vi "Puff_release3.vi"() -> (5 "Plug in titles":string[](array[string]), 7 "Plug in values":string[](array[string]))   [LabVIEW 2010]
uses:
  Controls/Post_Process.ctl
  Globals/Plug_in_data_global.vi
  Globals/Meas_global.vi
  Globals/Constants_global.vi
  Globals/Dynamic_call_global.ph.vi
  <vilib>/Analysis/NI_AALPro.lvlib
panel:
  in  "Save JPG images":bool
  out "delay":dbl format="%.2f"
  out "Pulse Width":dbl format="%.2f"
  out "falltime":dbl format="%.2f"
  out "top":dbl format="%.2f"
  out "risetime":dbl format="%.2f"
  in  "Save Time pdf?":bool
  out "Pdf":cluster{"Axis":dbl[], dbl[]}(graph)
  in  "Histogram Time":dbl format="%.2f"
  out "Current Block No":i32
  in  "Save averaged traces?":bool
  in  "Save Block Time Trace?":bool
  in  "Pause Mode":T1(ring)
  in  "OK":bool
  out "No of Valid Blocks":dbl
  out "Valve Trace":cluster{dbl, dbl, dbl[]}(graph)
  out "FFID Trace":cluster{dbl, dbl, dbl[]}(graph)
  out "Source On":i32
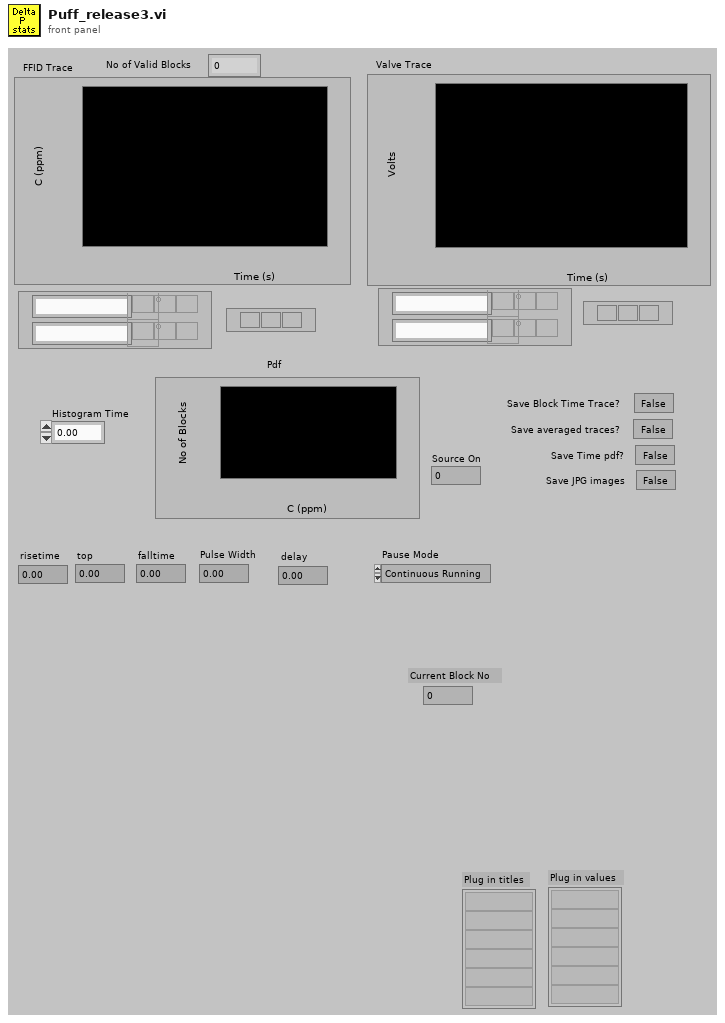
[diagram p1: front panel]
types:
  T1 = enum16{"Continuous Running", "After Each  Block"}
  T2 = typedef "Post_Process.ctl" = enum16{"Take New Data", "Post Process Raw Data File"}
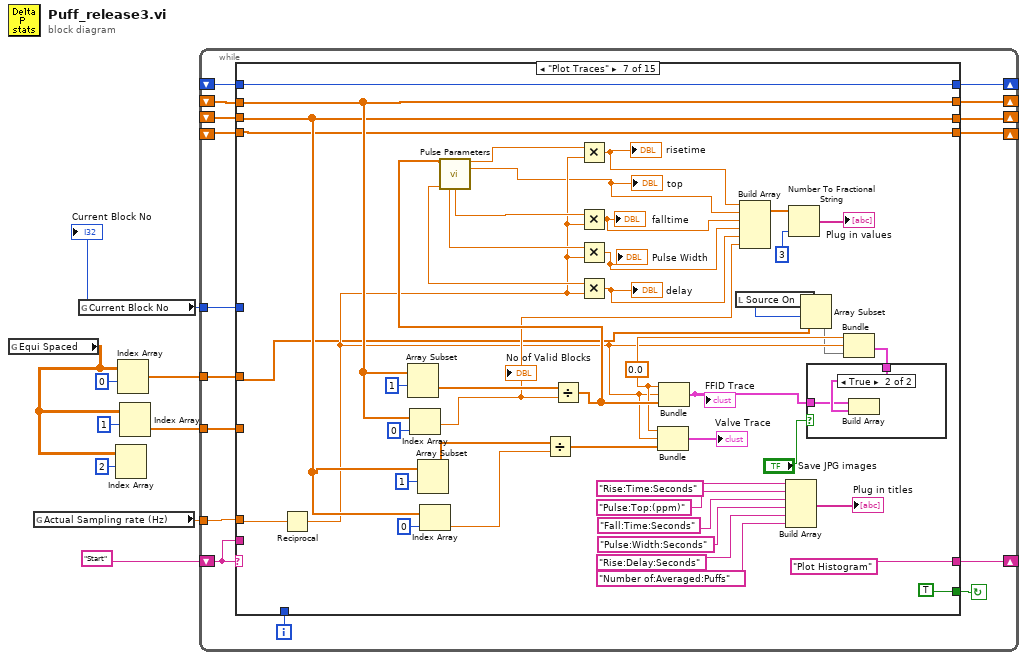
[diagram p0: block diagram]
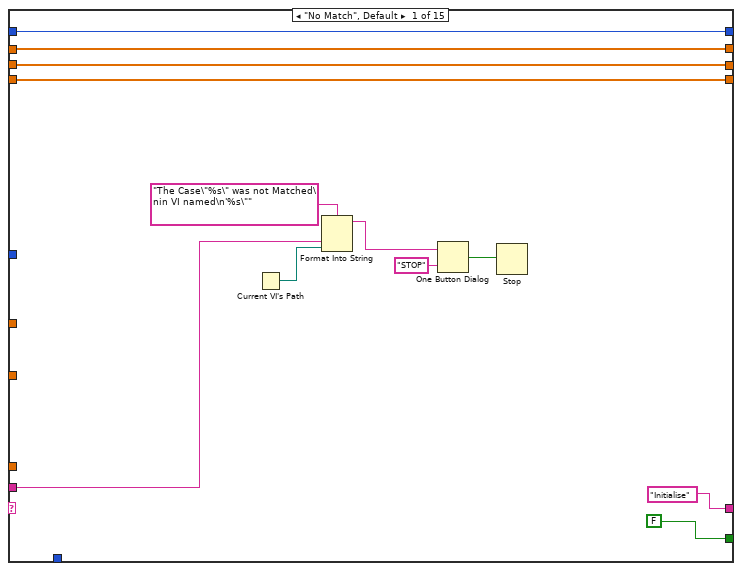
[diagram p2: hidden frame]
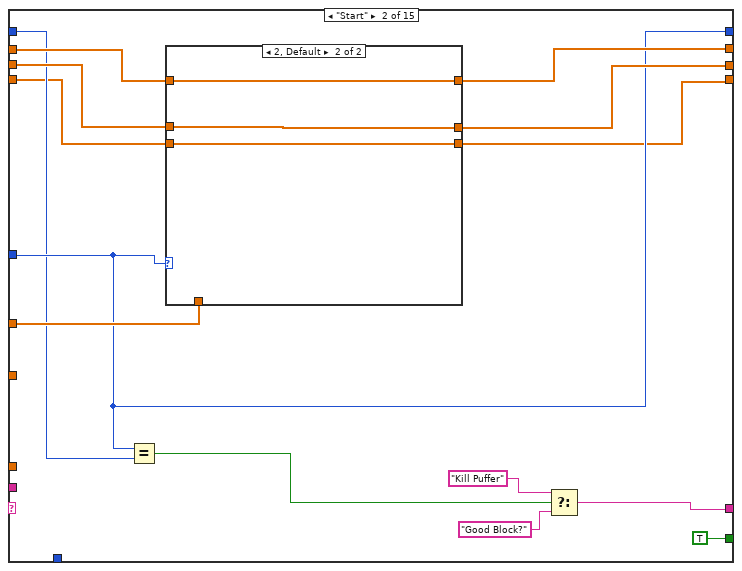
[diagram p3: hidden frame]
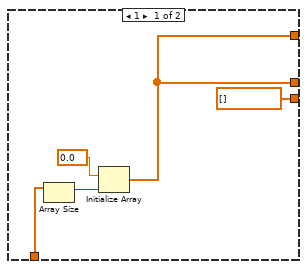
[diagram p4: hidden frame]
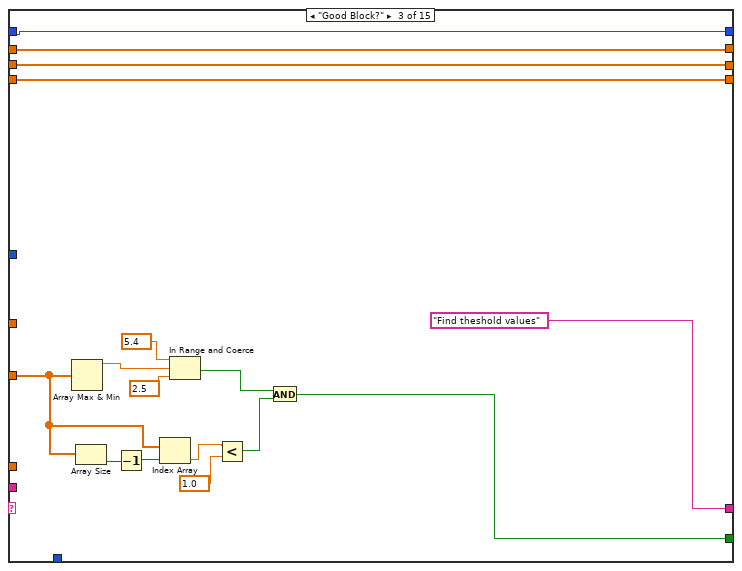
[diagram p5: hidden frame]
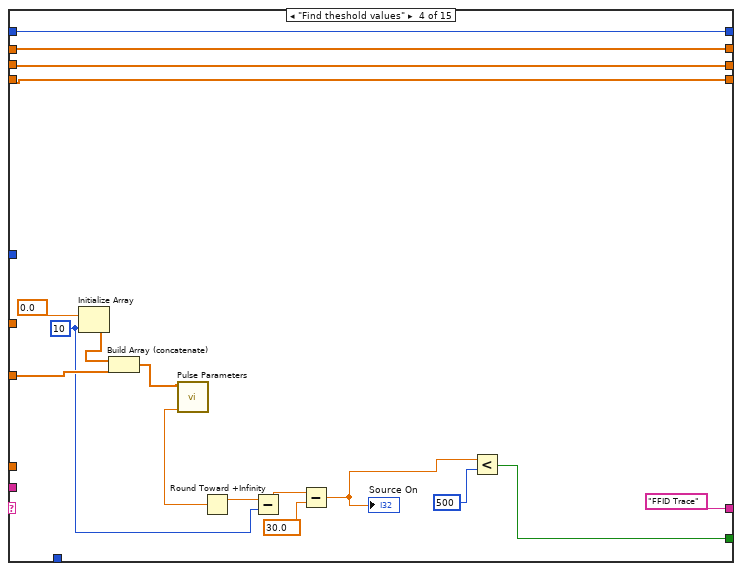
[diagram p6: hidden frame]
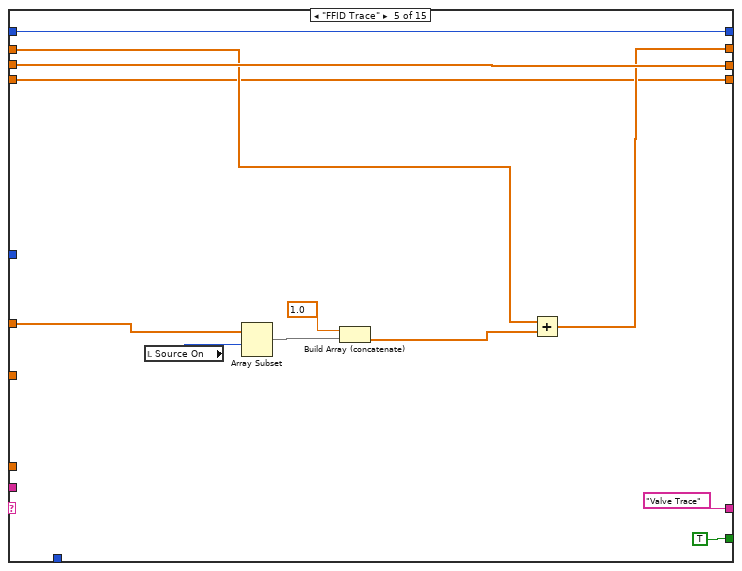
[diagram p7: hidden frame]
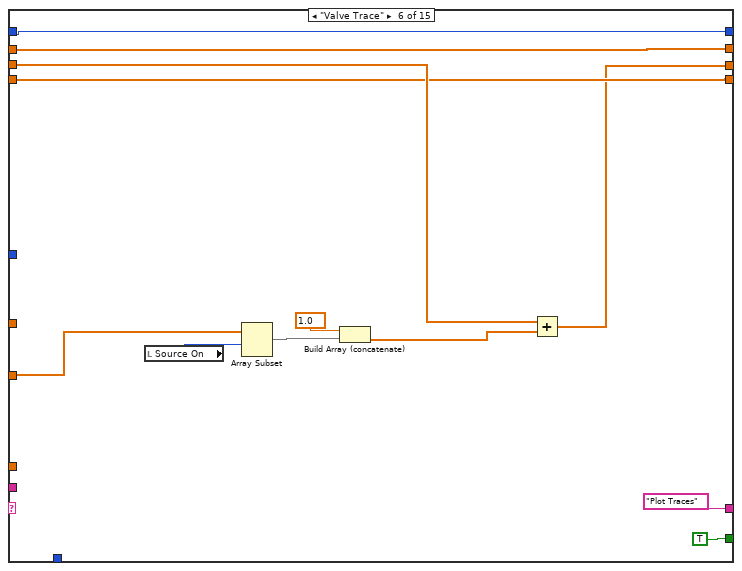
[diagram p8: hidden frame]
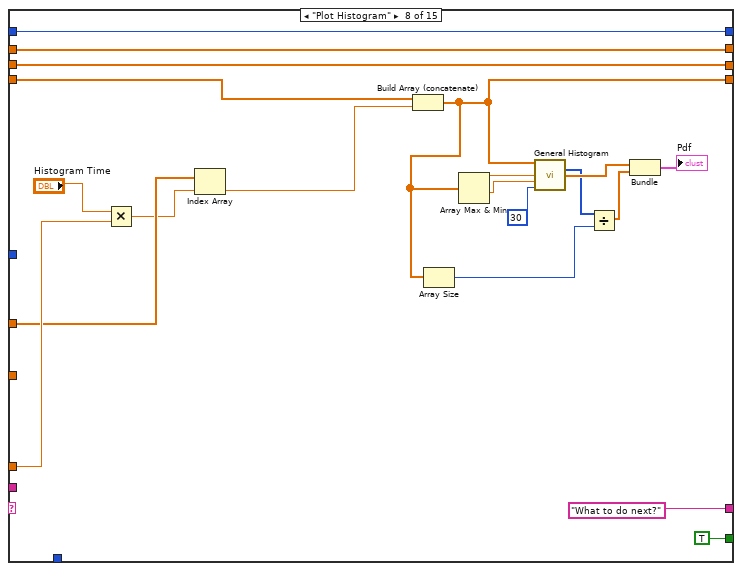
[diagram p10: hidden frame]
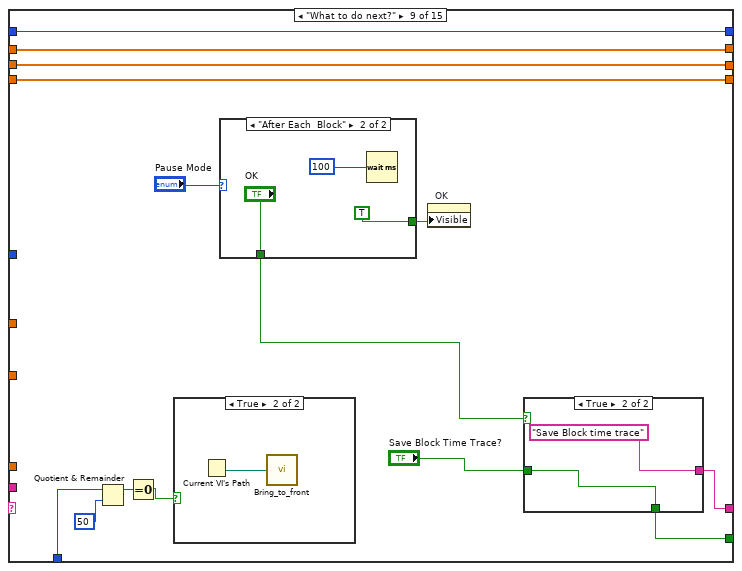
[diagram p11: hidden frame]
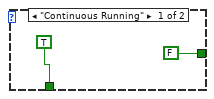
[diagram p13: hidden frame]
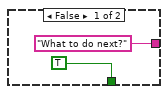
[diagram p14: hidden frame]
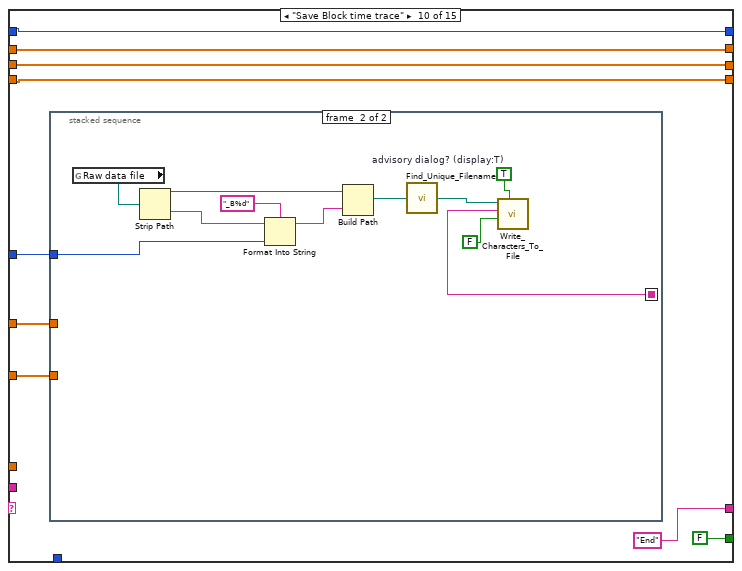
[diagram p15: hidden frame]
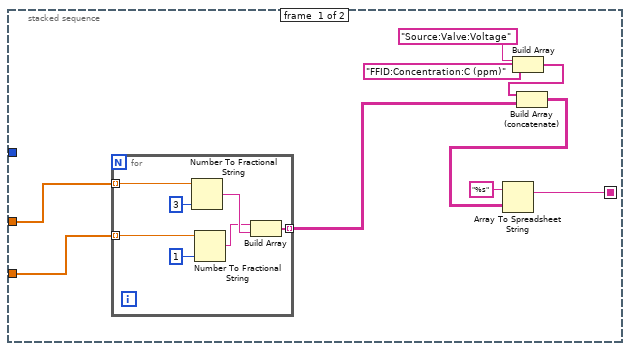
[diagram p16: hidden frame]
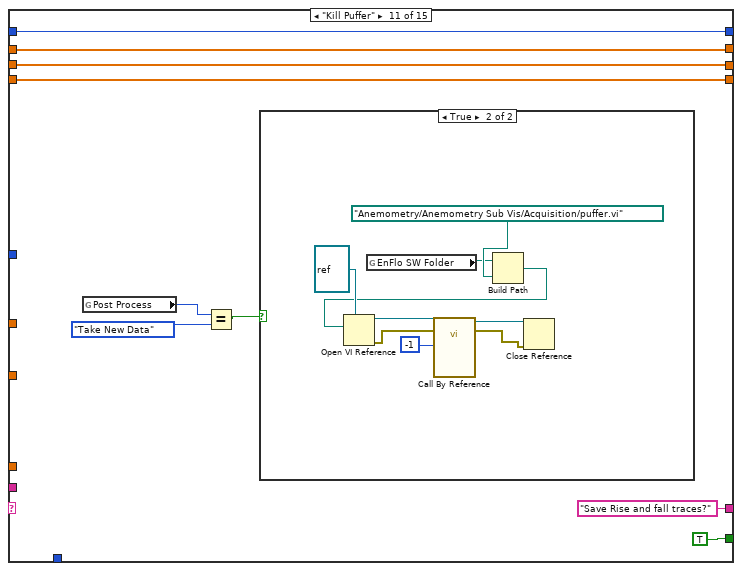
[diagram p17: hidden frame]
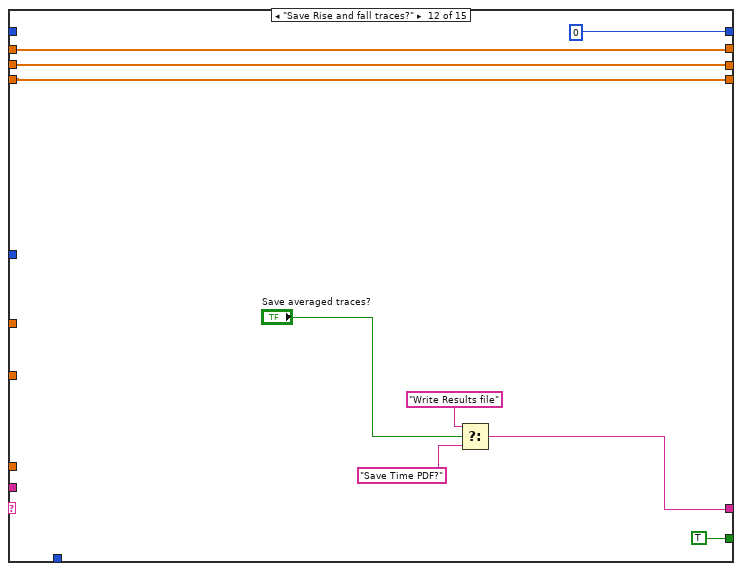
[diagram p19: hidden frame]
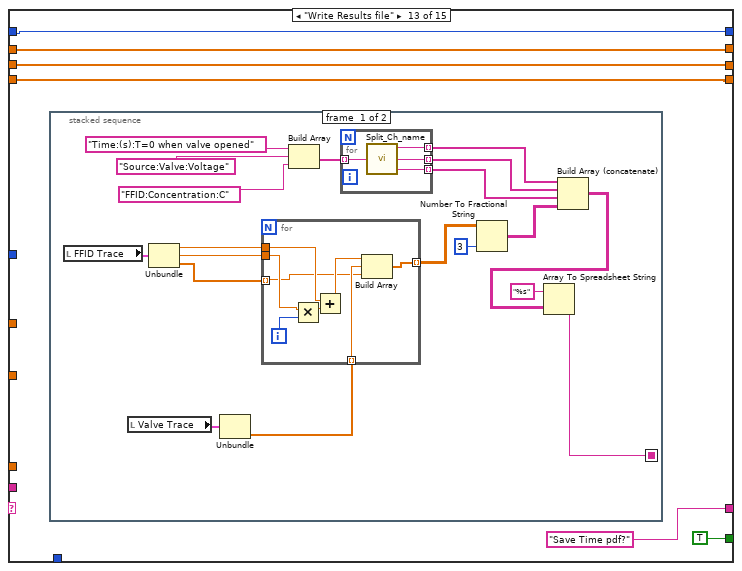
[diagram p20: hidden frame]
diagram:
  n1 = global read "Plug_in_data_global.vi" "Equi Spaced"() -> (w1:dbl[][])
  n2 = global read "Meas_global.vi" "Actual Sampling rate (Hz)"() -> (w5:dbl)
  n3 = global read "Meas_global.vi" "Current Block No"() -> (w4:i32)
  "Current Block No" <- w4
  n4 = Index Array(array=w1, index (row)=2) -> ()  [unwired: 1 in, 1 out]
  n5 = Index Array(array=w1, index (row)=0) -> (element=w6:dbl[])  [unwired: 1 in]
  n6 = Index Array(array=w1, index (row)=1) -> (element=w7:dbl[])  [unwired: 1 in]
  n7 = while {
    shift-left: "Start" -> [w23]
    shift-right: [w24] -> _
    shift-right: [w22] -> _
    shift-left: _ -> [w19]
    shift-right: [w21] -> _
    shift-left: _ -> [w20]
    tunnel: w7 -> [w18]
    tunnel: w6 -> [w17]
    tunnel: w5 -> [w16]
    tunnel: w4 -> [w15]
    shift-right: [w12] -> _
    shift-left: _ -> [w13]
    shift-right: [w10] -> _
    shift-left: _ -> [w11]
    i -> [w14]
    stop <- w25 continue-if-true
    n8 = case shown="\"Plot Traces\"" w23 {
      tunnel: [FALSE TRUE ("Processing last block?") w63 w88 TRUE ("Processing last block?") TRUE ("Processing last block?") TRUE ("Processing last block?") TRUE ("Processing last block?") w186 FALSE ("Processing last block?") TRUE ("Processing last block?") TRUE ("Processing last block?") TRUE ("Processing last block?") "Save Time pdf?" FALSE ("Processing last block?")] -> w25
      tunnel: ["Initialise" w41 "Find theshold values" "FFID Trace" "Valve Trace" "Plot Traces" "Plot Histogram" ("f") "What to do next?" ("f") w194 "End" "Save Rise and fall traces?" w263 "Save Time pdf?" "Save Time pdf" "End"] -> w24
      tunnel: w23 -> [w32 _ _ _ _ _ _ _ _ _ _ _ _ _ _]
      tunnel: [w29 w50 w75 w91 w100 w110 w159 w183 w197 w216 w252 w270 w276 w340 w349] -> w22
      tunnel: [w28 w48 w74 w90 w102 w105 w155 w182 w196 w215 w251 w269 w275 w339 w348] -> w21
      tunnel: w20 -> [w28 w47 w74 w90 w102 w109 w155 w182 w196 w215 w251 w269 w275 w339 w348]
      tunnel: w19 -> [w29 w49 w75 w91 w99 w110 w159 w183 w197 w216 w252 w270 w276 w340 w349]
      tunnel: w18 -> [_ _ w71 w84 _ w111 _ _ _ w212 _ _ _ _ w345]
      tunnel: w17 -> [_ w46 _ _ w101 _ w126 w178 _ w211 _ _ _ _ w344]
      tunnel: w16 -> [_ _ _ _ _ _ w151 w179 _ _ _ _ _ _ _]
      tunnel: w15 -> [_ w45 _ _ _ _ _ _ _ w210 _ _ _ _ w343]
      tunnel: w14 -> [_ _ _ _ _ _ _ _ w191 _ _ _ _ _ _]
      tunnel: w13 -> [w27 w44 w64 w87 w94 w108 w147 w181 w187 w209 w248 _ w272 _ w342]
      tunnel: [w27 w45 w64 w87 w94 w108 w147 w181 w187 w209 w248 0 w272 0 w342] -> w12
      tunnel: w11 -> [w26 w38 w62 w79 w93 w106 w130 w175 w184 w208 w244 w267 w271 w336 w341]
      tunnel: [w26 w39 w62 w79 w93 w106 w130 w167 w184 w208 w244 w267 w271 w336 w341] -> w10
      frame "No Match", Default {
        n9 = Current VI's Path() -> (path=w31:path)
        n10 = Format Into String(format string="The Case\"%s\" was not Matched\nin VI named\n'%s\"" ("Format String"), w32, w31) -> (resulting string=w35:string)  [unwired: 2 in, 1 out]
        n11 = One Button Dialog(message=w35, button name ("OK")="STOP") -> (true=w33:bool)
        n12 = Stop(stop? (T)=w33) -> ()
      }
      frame "Start" {
        n13 = Equal?(x=w45, y=w44) -> (x = y?=w43:bool)
        n14 = case shown="2, Default" w45 {
          tunnel: [w53 w59] -> w50
          tunnel: w49 -> [_ w59]
          tunnel: [w53 w58] -> w48
          tunnel: w47 -> [_ w58]
          tunnel: w46 -> [w56 _]
          tunnel: [dbl[] [] w57] -> w39
          tunnel: w38 -> [_ w57]
          frame 1 {
            n15 = Array Size(array=w56) -> (size(s)=w55:i32)
            n16 = Initialize Array(0.0 ("element"), w55) -> (w53:dbl[])
          }
          frame 2, Default {
          }
        }
        n17 = Select(t="Kill Puffer", s=w43, f="Good Block?") -> (s? t:f=w41:string)
      }
      frame "Good Block?" {
        n18 = Array Max & Min(array=w71) -> (max value=w61:dbl)  [unwired: 3 out]
        n19 = Array Size(array=w71) -> (size(s)=w70:i32)
        n20 = Decrement(x=w70) -> (x-1=w69:i32)
        n21 = Index Array(array=w71, index=w69) -> (element=w68:dbl)
        n22 = In Range and Coerce(upper limit=5.4, x=w61, lower limit=2.5 ("y")) -> (In Range?=w65:bool)  [unwired: 1 out]
        n23 = Less?(x=w68, y=1.0) -> (x < y?=w66:bool)
        n24 = And(x=w65, y=w66) -> (x .and. y?=w63:bool)
      }
      frame "Find theshold values" {
        w80 = 10 ("dimension size")
        n25 = Initialize Array(0.0, w80) -> (w83:dbl[])
        n26 = Build Array (concatenate)(w83, w84) -> (w85:dbl[])
        n27 = call <vilib>:"Pulse Parameters.vi"("X"=w85) -> ("delay"=w82:dbl)  [unwired: 4 in, 10 out]
        n28 = Round Toward +Infinity(x=w82) -> (ceil(x): smallest int >= x=w81:dbl)
        n29 = Subtract(x=w81, y=w80) -> (x-y=w78:dbl)
        n30 = Subtract(x=w78, y=30.0) -> (x-y=w76:dbl)
        "Source On" <- w76
        n31 = Less?(x=w76, y=500) -> (x < y?=w88:bool)
      }
      frame "FFID Trace" {
        n32 = local read "Source On"() -> (w96:i32)
        n33 = Array Subset(array=w101, index=w96) -> (w95:dbl[])  [unwired: 1 in]
        n34 = Build Array (concatenate)(1.0, w95) -> (w97:dbl[])
        n35 = Add(x=w99, y=w97) -> (x+y=w100:dbl[])
      }
      frame "Valve Trace" {
        n36 = local read "Source On"() -> (w113:i32)
        n37 = Array Subset(array=w111, index=w113) -> (w112:dbl[])  [unwired: 1 in]
        n38 = Build Array (concatenate)(1.0, w112) -> (w114:dbl[])
        n39 = Add(x=w109, y=w114) -> (x+y=w105:dbl[])
      }
      frame "Plot Traces" {
        w129 = 0.0
        n40 = Reciprocal(x=w151) -> (1/x=w128:dbl)
        n41 = Array Subset(array=w159, index=1) -> (w158:dbl[])  [unwired: 1 in]
        n42 = Index Array(array=w159, index=0) -> (element=w138:dbl)
        "No of Valid Blocks" <- w138
        n43 = Array Subset(array=w155, index=1) -> (w154:dbl[])  [unwired: 1 in]
        n44 = Index Array(array=w155, index=0) -> (element=w153:dbl)
        n45 = Divide(x=w154, y=w153) -> (x/y=w149:dbl[])
        n46 = Divide(x=w158, y=w138) -> (x/y=w146:dbl[])
        n47 = call <vilib>:"Pulse Parameters.vi"("X"=w146) -> ("risetime"=w145:dbl, "top"=w122:dbl, "delay"=w142:dbl, "duration"=w143:dbl, "falltime"=w144:dbl)  [unwired: 4 in, 6 out]
        "top" <- w122
        n48 = Multiply(x=w145, y=w128) -> (x*y=w121:dbl)
        "risetime" <- w121
        n49 = Multiply(x=w144, y=w128) -> (x*y=w120:dbl)
        "falltime" <- w120
        n50 = Multiply(x=w143, y=w128) -> (x*y=w119:dbl)
        "Pulse Width" <- w119
        n51 = Multiply(x=w142, y=w128) -> (x*y=w118:dbl)
        "delay" <- w118
        n52 = Bundle(w129, w128, w149) -> (→"Valve Trace":cluster{dbl, dbl, dbl[]})  [unwired: 1 in]
        n53 = Bundle(w129, w128, w146) -> (w123:cluster{dbl, dbl, dbl[]})  [unwired: 1 in]
        "FFID Trace" <- w123
        n54 = local read "Source On"() -> (w127:i32)
        n55 = Build Array(w121, w122, w120, w119, w118, w138) -> (w141:dbl[])
        n56 = Build Array("Rise:Time:Seconds", "Pulse:Top:(ppm)", "Fall:Time:Seconds", "Pulse:Width:Seconds", "Rise:Delay:Seconds", "Number of:Averaged:Puffs") -> (→"Plug in titles":string[])
        n57 = Number To Fractional String(number=w141, precision (6)=i16 3) -> (F-format string=→"Plug in values":string[])  [unwired: 2 in]
        n58 = Array Subset(array=w126, index=w127) -> (w125:dbl[])  [unwired: 1 in]
        n59 = Bundle(w129, w128, w125) -> (w124:cluster{dbl, dbl, dbl[]})  [unwired: 1 in]
        n60 = case shown="True" "Save JPG images" {
          tunnel: w124 -> [_ w163]
          tunnel: w123 -> [_ w162]
          frame False {
          }
          frame True {
            n61 = Build Array(w162, w163) -> ()  [unwired: 1 out]
          }
        }
      }
      frame "Plot Histogram" {
        n62 = Multiply(x="Histogram Time", y=w179) -> (x*y=w177:dbl)
        n63 = Index Array(array=w178, index=w177) -> (element=w176:dbl)
        n64 = Build Array (concatenate)(w175, w176) -> (w167:dbl[])
        n65 = Array Size(array=w167) -> (size(s)=w165:i32)
        n66 = Array Max & Min(array=w167) -> (max value=w174:dbl, min value=w173:dbl)  [unwired: 2 out]
        n67 = call <vilib>:"General Histogram.vi"("X"=w167, "max"=w174, "min"=w173, "# bins"=30) -> ("Histogram"=w166:i32[], "Axis"=w171:dbl[])  [unwired: 7 in, 3 out]
        n68 = Divide(x=w166, y=w165) -> (x/y=w164:dbl[])
        n69 = Bundle("Axis"=w171, w164) -> (→"Pdf":cluster{"Axis":dbl[], dbl[]})  [unwired: 1 in]
      }
      frame "What to do next?" {
        n70 = Quotient & Remainder(x=w191, y=50) -> (x-y*floor(x/y)=w189:i32)  [unwired: 1 out]
        n71 = Equal To 0?(x=w189) -> (x = 0?=w188:bool)
        n72 = case shown="True" w188 {
          frame False {
          }
          frame True {
            n73 = Current VI's Path() -> (path=w198:path)
            n74 = call "Bring_to_front.vi"("path"=w198) -> ()
          }
        }
        n75 = case shown="\"After Each  Block\"" "Pause Mode" {
          tunnel: [TRUE "OK"] -> w185
          tunnel: [FALSE TRUE] -> w192
          frame "Continuous Running" {
          }
          frame "After Each  Block" {
            n76 = Wait (ms)(milliseconds to wait=u32 100 ("f")) -> ()  [unwired: 1 out]
          }
        }
        n77 = property on="OK" class="Bool"("Visible"=w192) -> ()  [unwired: 2 in, 2 out]
        n78 = case shown="True" w185 {
          tunnel: "Save Block Time Trace?" -> [_ w206]
          tunnel: ["What to do next?" "Save Block time trace" ("t")] -> w194
          tunnel: [TRUE ("Processing last block?") w206] -> w186
          frame False {
          }
          frame True {
          }
        }
      }
      frame "Save Block time trace" {
        n79 = stacked-sequence {
          seq-local: [w220 _] -> [_ w238]
          tunnel: w212 -> [w219 _]
          tunnel: w211 -> [w218 _]
          tunnel: w210 -> [_ w235]
          frame #0 {
            n80 = for {
              tunnel: w219 -> [w230] mode=indexing
              tunnel: w218 -> [w229] mode=indexing
              tunnel: [w228] -> w217 mode=indexing
              n81 = Number To Fractional String(number=w229, precision (6)=i16 3) -> (F-format string=w227:string)  [unwired: 2 in]
              n82 = Number To Fractional String(number=w230, precision (6)=i16 1) -> (F-format string=w226:string)  [unwired: 2 in]
              n83 = Build Array(w226, w227) -> (w228:string[])
            }
            n84 = Build Array("Source:Valve:Voltage", "FFID:Concentration:C (ppm)") -> (w223:string[])
            n85 = Build Array (concatenate)(w223, w217) -> (w222:string[][])
            n86 = Array To Spreadsheet String(array=w222, 3:"%s" ("format string")) -> (spreadsheet string=w220:string)  [unwired: 1 in]
          }
          frame #1 {
            w240 = TRUE  # advisory dialog? (display:T)
            n87 = global read "Meas_global.vi" "Raw data file"() -> (w243:path)
            n88 = Strip Path(path=w243) -> (stripped path=w237:path, name=w236:string)
            n89 = Format Into String(format string="_B%d", initial string=w236, w235) -> (resulting string=w233:string)  [unwired: 1 in, 1 out]
            n90 = Build Path(base path=w237, name or relative path=w233) -> (appended path=w242:path)
            n91 = call "Find_Unique_Filename.vi"("Path In"=w242) -> ("Unique Path Out"=w241:path)  [unwired: 2 in]
            n92 = call "Write_Characters_To_File.vi"("file path (dialog if empty)"=w241, "advisory dialog? (display:T)"=w240, "character string"=w238, "append to file? (new file:F)"=FALSE) -> ()  [unwired: 4 in, 1 out]
          }
        }
      }
      frame "Kill Puffer" {
        n93 = global read "Meas_global.vi" "Post Process"() -> (w247:T2)
        n94 = Equal?(x=w247, y=Post_Process."Take New Data" ("Post Process")) -> (x = y?=w245:bool)
        n95 = case shown="True" w245 {
          frame False {
          }
          frame True {
            n96 = global read "Constants_global.vi" "EnFlo SW Folder"() -> (w253:path)
            n97 = Build Path(base path=w253, name or relative path=path "Anemometry/Anemometry Sub Vis/Acquisition/puffer.vi") -> (appended path=w255:path)
            n98 = Open VI Reference(type specifier VI Refnum (for type only)=refnum<vi> refnum, vi path=w255) -> (vi reference=w256:refnum<vi>, error out=w260:errorcluster)  [unwired: 4 in]
            n99 = call-by-ref "?"(reference=w256, error in=w260, "number of puffs (cont:0, stop:-1)"=-1) -> (reference out=w259:refnum<vi>, error out=w261:errorcluster)  [unwired: 2 in, 2 out]
            n100 = Close Reference(reference=w259, error in (no error)=w261) -> ()  [unwired: 1 out]
          }
        }
      }
      frame "Save Rise and fall traces?" {
        n101 = Select(t="Write Results file", s="Save averaged traces?", f="Save Time PDF?") -> (s? t:f=w263:string)
      }
      frame "Write Results file" {
        n102 = stacked-sequence {
          seq-local: [w285 _] -> [_ w309]
          frame #0 {
            n103 = local read "FFID Trace"() -> (w295:cluster{dbl, dbl, dbl[]})
            n104 = local read "Valve Trace"() -> (w284:cluster{dbl, dbl, dbl[]})
            n105 = Unbundle(w295) -> (w293:dbl, w294:dbl, w292:dbl[])
            n106 = Unbundle(w284) -> (w283:dbl[])  [unwired: 2 out]
            n107 = for {
              tunnel: w294 -> [w306]
              tunnel: w293 -> [w305]
              tunnel: w292 -> [w300] mode=indexing
              tunnel: [w303] -> w290 mode=indexing
              tunnel: w283 -> [w301] mode=indexing
              i -> [w307]
              n108 = Multiply(x=w306, y=w307) -> (x*y=w304:dbl)
              n109 = Add(x=w305, y=w304) -> (x+y=w302:dbl)
              n110 = Build Array(w302, w301, w300) -> (w303:dbl[])
            }
            n111 = Build Array("Time:(s):T=0 when valve opened", "Source:Valve:Voltage", "FFID:Concentration:C") -> (w280:string[])
            n112 = for {
              tunnel: w280 -> [w299] mode=indexing
              tunnel: [w298] -> w279 mode=indexing
              tunnel: [w297] -> w278 mode=indexing
              tunnel: [w296] -> w277 mode=indexing
              n113 = call "Split_Ch_name.vi"("Ch name"=w299) -> ("Top level"=w298:string, "Middle"=w297:string, "Low level"=w296:string)
            }
            n114 = Number To Fractional String(number=w290, precision (6)=i16 3) -> (F-format string=w289:string[][])  [unwired: 2 in]
            n115 = Build Array (concatenate)(w279, w278, w277, w289) -> (w287:string[][])
            n116 = Array To Spreadsheet String(array=w287, 3:"%s" ("format string")) -> (spreadsheet string=w285:string)  [unwired: 1 in]
          }
          frame #1 {
            w325 = TRUE  # advisory dialog? (display:T)
            n117 = global read "Dynamic_call_global.ph.vi" "Plug in titles"() -> (w321:string[])
            n118 = global read "Dynamic_call_global.ph.vi" "Plug in values"() -> (w317:string[])
            n119 = global read "Meas_global.vi" "Raw data file"() -> (w330:path)
            n120 = Strip Path(path=w330) -> (stripped path=w322:path, name=w323:string)
            n121 = for {
              tunnel: w321 -> [w334] mode=indexing
              tunnel: [w333] -> w320 mode=indexing
              tunnel: [w332] -> w319 mode=indexing
              tunnel: [w331] -> w318 mode=indexing
              n122 = call "Split_Ch_name.vi"("Ch name"=w334) -> ("Top level"=w333:string, "Middle"=w332:string, "Low level"=w331:string)
            }
            n123 = Concatenate Strings(w323, "_P" ("string")) -> (w329:string)
            n124 = Initialize Array("", 15) -> (w314:string[])
            n125 = Build Path(base path=w322, name or relative path=w329) -> (appended path=w327:path)
            n126 = call "Asterisk_header.vi"("Channel names"=w314) -> ("Header string"=w310:string)
            n127 = call "Find_Unique_Filename.vi"("Path In"=w327) -> ("Unique Path Out"=w326:path)  [unwired: 2 in]
            n128 = Build Array(w320, w319, w318, w317) -> (w315:string[][])
            n129 = Array To Spreadsheet String(array=w315, 3:"%s" ("format string")) -> (spreadsheet string=w311:string)  [unwired: 1 in]
            n130 = Concatenate Strings(w311, w310, w309) -> (w308:string)
            n131 = call "Write_Characters_To_File.vi"("file path (dialog if empty)"=w326, "advisory dialog? (display:T)"=w325, "character string"=w308, "append to file? (new file:F)"=FALSE) -> ()  [unwired: 4 in, 1 out]
          }
        }
      }
      frame "Save Time pdf?" {
      }
      frame "Save Time pdf" {
        n132 = stacked-sequence {
          seq-local: [w358 _] -> [_ w375]
          tunnel: w345 -> [_ _]
          tunnel: w344 -> [_ _]
          tunnel: w343 -> [_ _]
          frame #0 {
            n133 = local read "Pdf"() -> (w356:cluster{"Axis":dbl[], dbl[]})
            n134 = Unbundle(w356) -> ("Axis"=w355:dbl[], w354:dbl[])
            n135 = for {
              tunnel: w354 -> [w372] mode=indexing
              tunnel: w355 -> [w371] mode=indexing
              tunnel: [w370] -> w357 mode=indexing
              n136 = Number To Fractional String(number=w372, precision (6)=i16 3) -> (F-format string=w368:string)  [unwired: 2 in]
              n137 = Number To Fractional String(number=w371, precision (6)=i16 3) -> (F-format string=w369:string)  [unwired: 2 in]
              n138 = Build Array(w369, w368) -> (w370:string[])
            }
            n139 = Build Array("FFID:Concentration:C (ppm)", "Pdf:Bin:Frequency") -> (w353:string[])
            n140 = for {
              tunnel: w353 -> [w366] mode=indexing
              tunnel: [w365] -> w352 mode=indexing
              tunnel: [w364] -> w351 mode=indexing
              tunnel: [w363] -> w350 mode=indexing
              n141 = call "Split_Ch_name.vi"("Ch name"=w366) -> ("Top level"=w365:string, "Middle"=w364:string, "Low level"=w363:string)
            }
            n142 = Build Array (concatenate)(w352, w351, w350, w357) -> (w360:string[][])
            n143 = Array To Spreadsheet String(array=w360, 3:"%s" ("format string")) -> (spreadsheet string=w358:string)  [unwired: 1 in]
          }
          frame #1 {
            w394 = TRUE  # advisory dialog? (display:T)
            n144 = global read "Dynamic_call_global.ph.vi" "Plug in titles"() -> (w387:string[])
            n145 = global read "Dynamic_call_global.ph.vi" "Plug in values"() -> (w383:string[])
            n146 = global read "Meas_global.vi" "Raw data file"() -> (w397:path)
            n147 = local read "Histogram Time"() -> (w388:dbl)
            n148 = Strip Path(path=w397) -> (stripped path=w392:path, name=w391:string)
            n149 = for {
              tunnel: w387 -> [w401] mode=indexing
              tunnel: [w400] -> w386 mode=indexing
              tunnel: [w399] -> w385 mode=indexing
              tunnel: [w398] -> w384 mode=indexing
              n150 = call "Split_Ch_name.vi"("Ch name"=w401) -> ("Top level"=w400:string, "Middle"=w399:string, "Low level"=w398:string)
            }
            n151 = Format Into String(format string="_T=%.2f", initial string=w391, w388) -> (resulting string=w389:string)  [unwired: 1 in, 1 out]
            n152 = Initialize Array("", 15) -> (w380:string[])
            n153 = Build Path(base path=w392, name or relative path=w389) -> (appended path=w396:path)
            n154 = call "Asterisk_header.vi"("Channel names"=w380) -> ("Header string"=w376:string)
            n155 = call "Find_Unique_Filename.vi"("Path In"=w396) -> ("Unique Path Out"=w395:path)  [unwired: 2 in]
            n156 = Build Array(w386, w385, w384, w383) -> (w381:string[][])
            n157 = Array To Spreadsheet String(array=w381, 3:"%s" ("format string")) -> (spreadsheet string=w377:string)  [unwired: 1 in]
            n158 = Concatenate Strings(w377, w376, w375) -> (w374:string)
            n159 = call "Write_Characters_To_File.vi"("file path (dialog if empty)"=w395, "advisory dialog? (display:T)"=w394, "character string"=w374, "append to file? (new file:F)"=FALSE) -> ()  [unwired: 4 in, 1 out]
          }
        }
      }
    }
  }
